vi "ToSTM.vi"(7 "error in (no error)":errorcluster, 8 "Servo position":string, 9 "Baud rate":u32=115200, 10 "Serial port":refnum<visa-resource-name>="COM6") -> (0 "error out":errorcluster, 2 "Feedback message":string)   [LabVIEW 2020]
doc: "This VI sends <B>Servo position</B> to serial port and returns feedback message.\nTo communicate correctly, you need to choose which <B>Serial Port</B> your device is connected and what <B>Baud Rate</B> it runs.\nRemember, that after sending Servo position, you need to return Feedback message from device."
uses:
  <vilib>/Instr/_visa.llb/VISA Configure Serial Port (Instr).vi
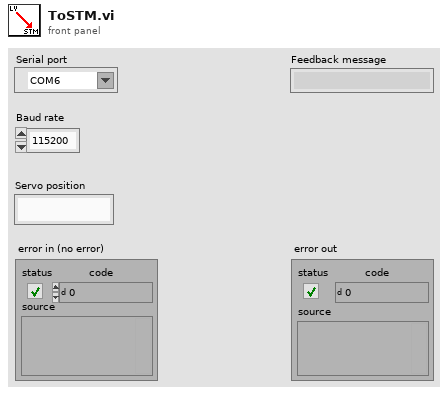
[diagram p1: front panel]
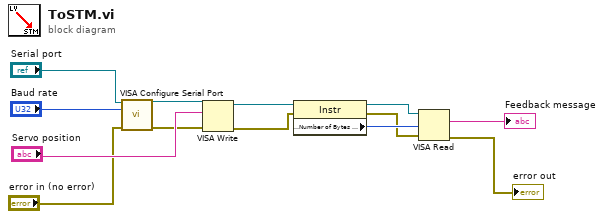
[diagram p0: block diagram]
diagram:
  n1 = call-poly "VISA Configure Serial Port"("VISA resource name"="Serial port", "baud rate (9600)"="Baud rate", "error in (no error)"="error in (no error)") -> ("VISA resource name out"=w10:refnum<visa-resource-name>, "error out"=w2:errorcluster)  [unwired: 11 in]
  n2 = VISA Write(VISA resource name=w10, write buffer="Servo position", error in (no error)=w2) -> (VISA resource name out=w11:refnum<visa-resource-name>, error out=w5:errorcluster)  [unwired: 1 out]
  n3 = property class="Instr"(reference=w11, error in=w5) -> (reference out=w12:refnum<visa-resource-name>, error out=w4:errorcluster, "Serial Settings:Number of Bytes at Serial Port"=w13:u32)
  n4 = VISA Read(VISA resource name=w12, byte count=w13, error in (no error)=w4) -> (read buffer=→"Feedback message":string, error out=→"error out":errorcluster)  [unwired: 2 out]
